vi "Set output map.vi"(4 "Map":cluster{"CobID":u32, "nBytes":u8}[](array[cluster]), 7 "CANopen in":refnum<class "CANopen.lvclass">) -> (3 "CANopen out":refnum<class "CANopen.lvclass">)   [LabVIEW 2026, in "canopen_.lvlib" / "CANopen.lvclass"]
doc: "Sets the map table to use for the outputs (usually RxPDO messages). Check \"CAN output\" for details on how the output map is used."
uses:
  CANopen.lvclass
  CANopen.lvclass/CANopen.ctl
panel:
  out "Output image":u8[](array[numeric])
  out "Output map":cluster{"CobID":u32, "nBytes":u8}[](array[cluster])
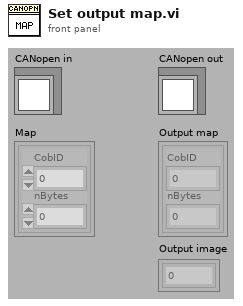
[diagram p1: front panel]
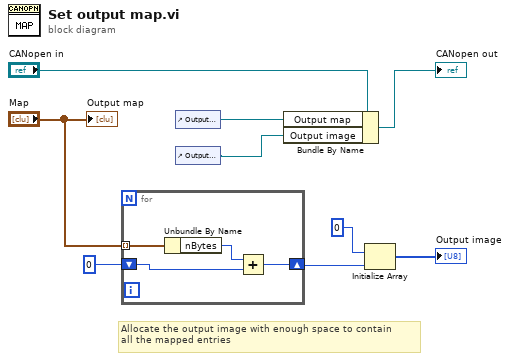
[diagram p0: block diagram]
diagram:
  # "Allocate the output image with enough space to contain\nall the mapped entries"
  n1 = for {
    tunnel: "Map" -> [w13] mode=indexing
    shift-right: [w10] -> w6
    shift-left: u16 0 -> [w11]
    n2 = Unbundle By Name(w13) -> ("nBytes"=w12:u8)
    n3 = Add(x=w12, y=w11) -> (x+y=w10:u16)
  }
  n4 = control-ref of="Output map"() -> (w4:refnum<vi>)
  n5 = control-ref of="Output image"() -> (w1:refnum<vi>)
  n6 = Bundle By Name(cluster="CANopen in", "Output map"=w4, "Output image"=w1) -> (→"CANopen out":refnum<class "CANopen.lvclass">)
  n7 = Initialize Array(u8 0 ("nBytes"), w6) -> (→"Output image":u8[])
  "Output map" <- "Map"
